vi "Get Type.vi"(8 "error in (no error)":errorcluster caption="Error In", 11 "Path In":path) -> (0 "error out":errorcluster caption="Error Out", 1 "Name":string, 2 "Enable?":bool, 3 "Driver Path":path)   [LabVIEW 2020]
uses:
  006 Path Management/006 Path.ctl
  <vilib>/Utility/file.llb/Read Delimited Spreadsheet (string).vi
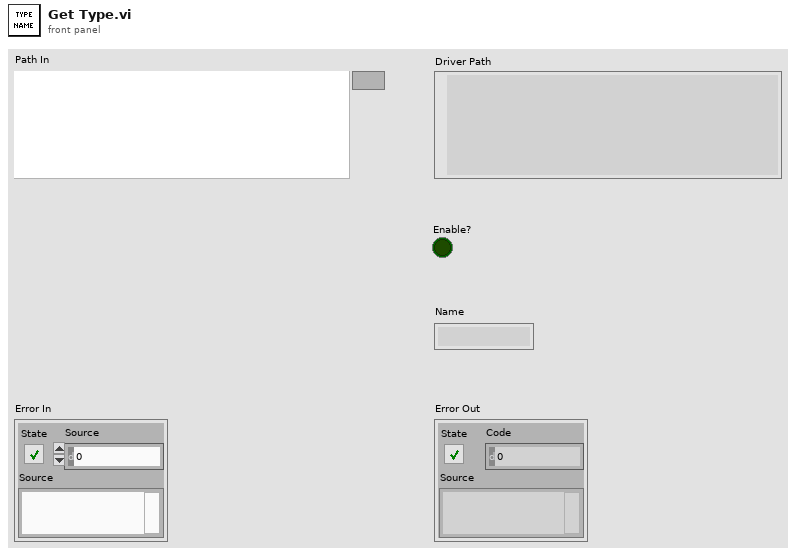
[diagram p1: front panel]
types:
  T1 = typedef "006 Path.ctl" = enum16{"Config", "Device.csv", "Version", "Project", "CertainProject", "Project Info.xml", "00_DataSource", "01_DataGraph", "02_DataSave", "03_TestProcess", "04_DataUse", "00_Database.mdb", "01_DataModule.xml", "02_ControlPanel.xml", "02_ControlPanelData.xml", "03_FlowChart.xml", "03_FlowChartData.xml", "04_Parameter_Setting.xml", "04_ParameterSettingData.xml"}
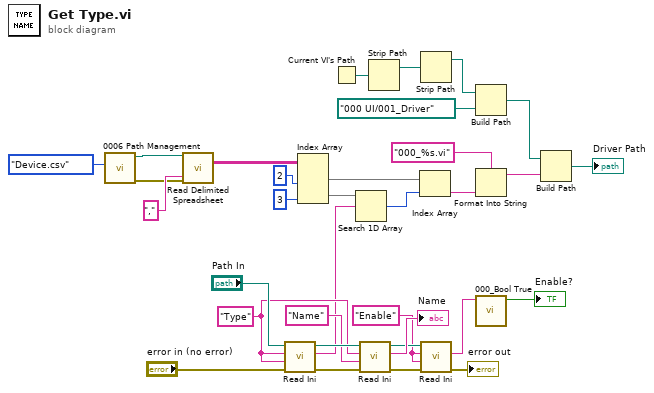
[diagram p0: block diagram]
diagram:
  w3 = "Enable" ("section")
  w29 = "Type" ("section")
  n1 = call "0006 Path Management.vi"("Path"=006_Path."Device.csv") -> ("error out"=w24:errorcluster, "Path Out"=w26:path)  [unwired: 8 in, 1 out]
  n2 = call-poly <vilib>:"Read Delimited Spreadsheet.vi"("file path (dialog if empty)"=w26, "error in (no error)"=w24, "delimiter (\\t)"="," ("delimiter (\\t)")) -> ("all rows"=w23:string[][])  [unwired: 7 in, 5 out]
  n3 = call "Read Ini.vi"("error in (no error)"="error in (no error)", "key"=w29, "section"=w29, "Path In"="Path In") -> ("error out"=w32:errorcluster, "value"=w16:string, "Path Out"=w31:path)  [unwired: 5 in]
  n4 = Index Array(array=w23, index (col) #1=2 ("禁用的索引 (列)"), index (col) #2=3 ("索引 (列)")) -> (element #1=w18:string[], element #2=w17:string[])  [unwired: 2 in]
  n5 = Current VI's Path() -> (path=w10:path)
  n6 = Search 1D Array(1D array=w17, element=w16) -> (index of element=w19:i32)  [unwired: 1 in]
  n7 = call "Read Ini.vi"("error in (no error)"=w32, "key"="Name", "section"=w29, "Path In"=w31) -> ("error out"=w5:errorcluster, "value"=→"Name":string, "Path Out"=w6:path)  [unwired: 5 in]
  n8 = Strip Path(path=w10) -> (stripped path=w11:path)  [unwired: 1 out]
  n9 = Index Array(array=w18, index=w19) -> (element=w14:string)
  n10 = Strip Path(path=w11) -> (stripped path=w12:path)  [unwired: 1 out]
  n11 = call "Read Ini.vi"("error in (no error)"=w5, "key"=w3, "section"=w3, "Path In"=w6) -> ("error out"=→"error out":errorcluster, "value"=w2:string)  [unwired: 5 in, 1 out]
  n12 = Build Path(base path=w12, name or relative path=path "000 UI/001_Driver" ("名称或相对路径")) -> (appended path=w9:path)
  n13 = Format Into String(format string="000_%s.vi" ("格式字符串"), w14) -> (resulting string=w7:string)  [unwired: 2 in, 1 out]
  n14 = call "000_Bool True.vi"("Bool String"=w2) -> ("True"=→"Enable?":bool)  [unwired: 9 in, 1 out]
  n15 = Build Path(base path=w9, name or relative path=w7) -> (appended path=→"Driver Path":path)
